vi "AvoidColision.vi"(0 "RobotRef":refnum<class "Robot.lvclass">[](array[class]), 2 "referencia":i32, 3 "positionOnWall":T1=enum."FrontWall", 5 "error in (no error)":errorcluster, 7 "Field":refnum<class "Field.lvclass">, 9 "robot Radius":dbl) -> (16 "dest_x":dbl, 17 "dest_y":dbl, 19 "error out":errorcluster)   [LabVIEW 2024, in "DefendAreaTactic.lvclass"]
uses:
  DefendAreaTactic.lvclass
  Robot_class/Robot.lvclass
  WallPositions.ctl
  Field_class/Field.lvclass
  Robot_class/Robot.lvclass/Robot.ctl
  Robot_class/Read dest_x.vi
  Robot_class/Read dest_y.vi
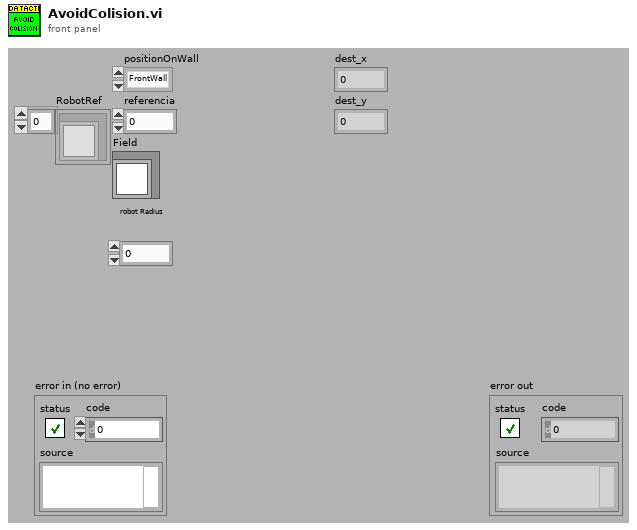
[diagram p1: front panel]
types:
  T1 = typedef "WallPositions.ctl" = enum16{"LeftWall", "LeftCorner", "FrontWall", "RightCorner", "RightWall"}
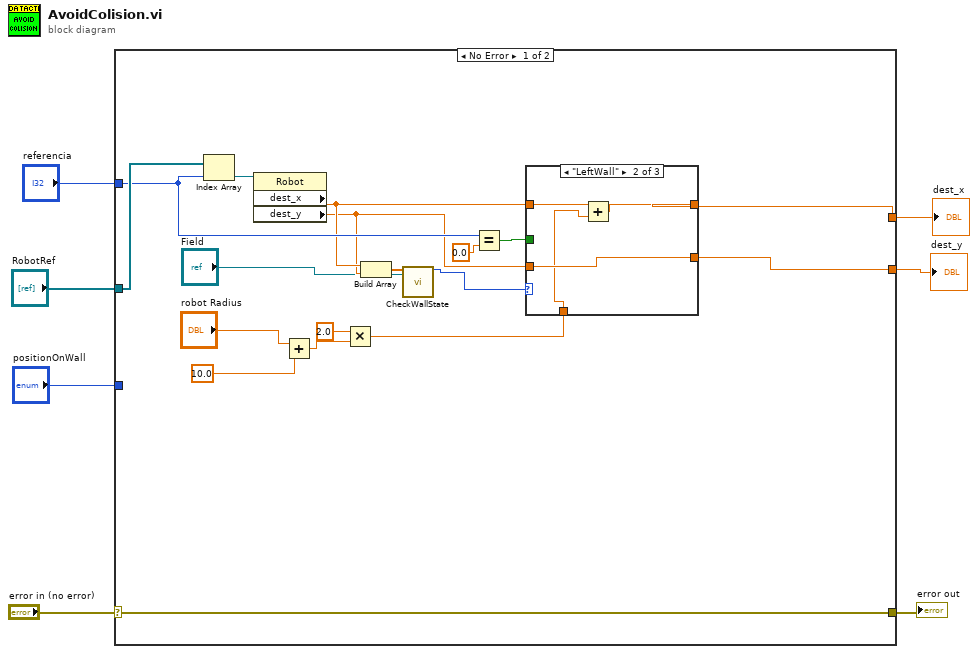
[diagram p0: block diagram]
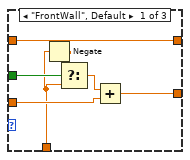
[diagram p2: hidden frame]
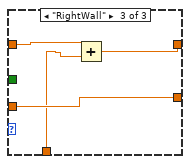
[diagram p3: hidden frame]
diagram:
  n1 = case shown="No Error" "error in (no error)" {
    selector: "error in (no error)" -> [w25 w41]
    tunnel: [w25 w41] -> w6
    tunnel: "RobotRef" -> [w24 _]
    tunnel: "positionOnWall" -> [_ _]
    tunnel: [w22 _] -> w3
    tunnel: [w21 _] -> w2
    tunnel: "referencia" -> [w18 _]
    frame No Error {
      n2 = Index Array(array=w24, index=w18) -> (element=w23:refnum<class "Robot.lvclass">)
      n3 = property class="Robot"(reference=w23) -> ("dest_x"=w12:dbl, "dest_y"=w11:dbl)  [unwired: 1 in, 2 out]
      n4 = Add(x="robot Radius", y=10.0) -> (x+y=w15:dbl)
      n5 = Multiply(x=2.0, y=w15) -> (x*y=w13:dbl)
      n6 = Build Array(w12, w11) -> (w10:dbl[])
      n7 = call "CheckWallState.vi"("Position"=w10, "Field"="Field") -> ("WallState"=w8:T1)  [unwired: 16 in, 1 out]
      n8 = Equal?(x=w18, y=0.0) -> (x = y?=w20:bool)
      n9 = case shown="\"LeftWall\"" w8 {
        tunnel: w12 -> [w32 w35 w40]
        tunnel: w11 -> [w29 w36 w38]
        tunnel: [w31 w36 w38] -> w21
        tunnel: [w32 w34 w39] -> w22
        tunnel: w20 -> [w28 _ _]
        tunnel: w13 -> [w27 w33 w37]
        frame "FrontWall", Default {
          n10 = Negate(x=w27) -> (-x=w26:dbl)
          n11 = Select(t=w26, s=w28, f=w27) -> (s? t:f=w30:dbl)
          n12 = Add(x=w30, y=w29) -> (x+y=w31:dbl)
        }
        frame "LeftWall" {
          n13 = Add(x=w35, y=w33) -> (x+y=w34:dbl)
        }
        frame "RightWall" {
          n14 = Add(x=w40, y=w37) -> (x+y=w39:dbl)
        }
      }
    }
    frame Error {
    }
  }
  "error out" <- w6
  "dest_x" <- w3
  "dest_y" <- w2
